vi "Write Acquisition  Enqueuer.vi"(8 "error in (no error)":errorcluster, 10 "Actor Framework:Message Enqueuer":refnum<class "Message Enqueuer.lvclass">, 11 "Grayscale in":refnum<class "Grayscale.lvclass">) -> (0 "error out":errorcluster, 3 "Grayscale out":refnum<class "Grayscale.lvclass">)   [LabVIEW 2015, in "Tests.lvlib" / "Grayscale.lvclass"]
uses:
  Grayscale.lvclass
  <vilib>/ActorFramework/Message Enqueuer/Message Enqueuer.lvclass
  Grayscale.lvclass/Grayscale.ctl
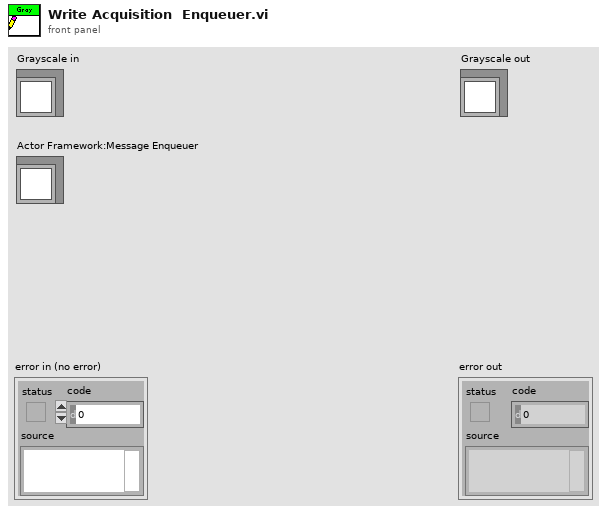
[diagram p1: front panel]
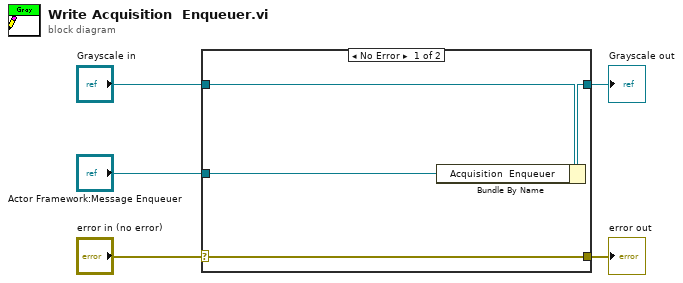
[diagram p0: block diagram]
diagram:
  n1 = case shown="No Error" "error in (no error)" {
    selector: "error in (no error)" -> [w9 w10]
    tunnel: [w9 w10] -> w4
    tunnel: [w7 w11] -> w2
    tunnel: "Grayscale in" -> [w8 w11]
    tunnel: "Actor Framework:Message Enqueuer" -> [w6 _]
    frame No Error {
      n2 = Bundle By Name(cluster=w8, "Acquisition  Enqueuer"=w6) -> (w7:refnum<class "Grayscale.lvclass">)
    }
    frame Error {
    }
  }
  "error out" <- w4
  "Grayscale out" <- w2
